vi "KalmanFilter_Predict.vi"(6 "dT_Seconds":dbl=0.02, 10 "U":T2, 11 "in KalmanFilter":T1) -> (0 "Error":bool, 3 "out KalmanFilter":T1)   [LabVIEW 2019, in "Trajectory_Library.lvlib"]
doc: "Creates a new LINEAR SYSTEM data cluster with the specified values. \n\n\nInputs: \n - XXX -- XXX.\n\nOutputs:\n - XXX -- XXX."
uses:
  Trajectory_Library.lvlib
  KALMAN_FILTER.ctl
  <vilib>/Analysis/Matrix/Datatypes/RealMatrix.ctl
  LINEAR_SYSTEM.ctl
  Discretization_DiscretizeAB.vi
  <vilib>/Analysis/baseanly.llb/A x B.vi
  <vilib>/Analysis/baseanly.llb/Real A x B.vi
  <vilib>/Analysis/7linalg.llb/Matrix Exp.vi
  <vilib>/Analysis/7linalg.llb/Real Matrix Exp.vi
  <vilib>/Analysis/Matrix/Numeric/Multiply/Multiply.vi
  <vilib>/Analysis/Matrix/Numeric/Multiply/Multiply - RM,R.vi
  <vilib>/Analysis/Matrix/Numeric/Add/Add.vi
  <vilib>/Analysis/Matrix/Numeric/Add/Add - RM,RM.vi
  <vilib>/Analysis/Matrix/NI_Matrix.lvlib
panel:
  # "<Inputs,1>"
  # "Steady State Gain  \n<States,Outputs>"
  # "State Estimate <Statess,1>"
  # "<States,States>"
  # "<States,Inputs>"
  # "<Outputs,States>"
  # "<Outputs,Inputs>"
  # "Steady State Gain  \n<States,Outputs>"
  # "State Estimate <Statess,1>"
  # "<States,States>"
  # "<States,Inputs>"
  # "<Outputs,States>"
  # "<Outputs,Inputs>"
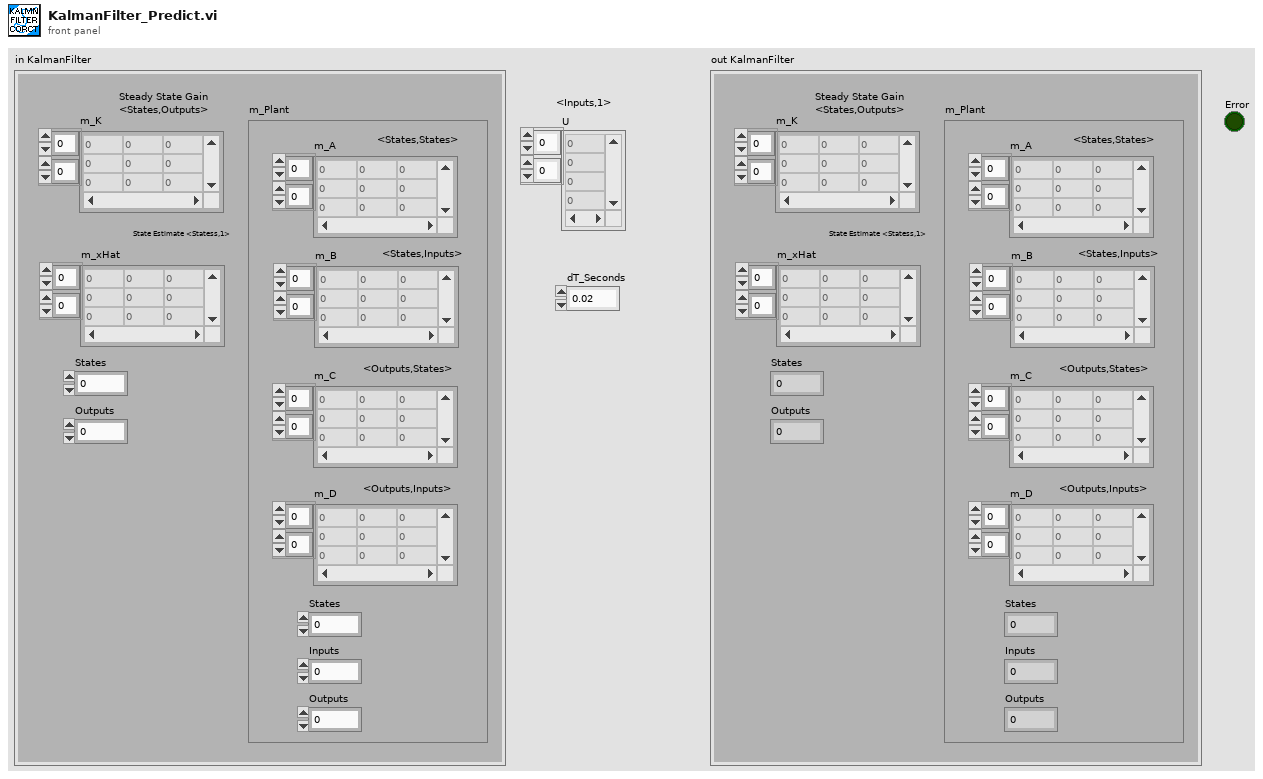
[diagram p1: front panel]
types:
  T1 = typedef "Trajectory_Library.lvlib/KALMAN_FILTER.ctl" = cluster{"m_K":T2, "m_xHat":T2, "States":i32, "Outputs":i32, "m_Plant":T3}
  T2 = typedef "NI_Matrix.lvlib/RealMatrix.ctl" = dbl[][]
  T3 = typedef "Trajectory_Library.lvlib/LINEAR_SYSTEM.ctl" = cluster{"m_A":T2, "m_B":T2, "m_C":T2, "m_D":T2, "States":i32, "Inputs":i32, "Outputs":i32}
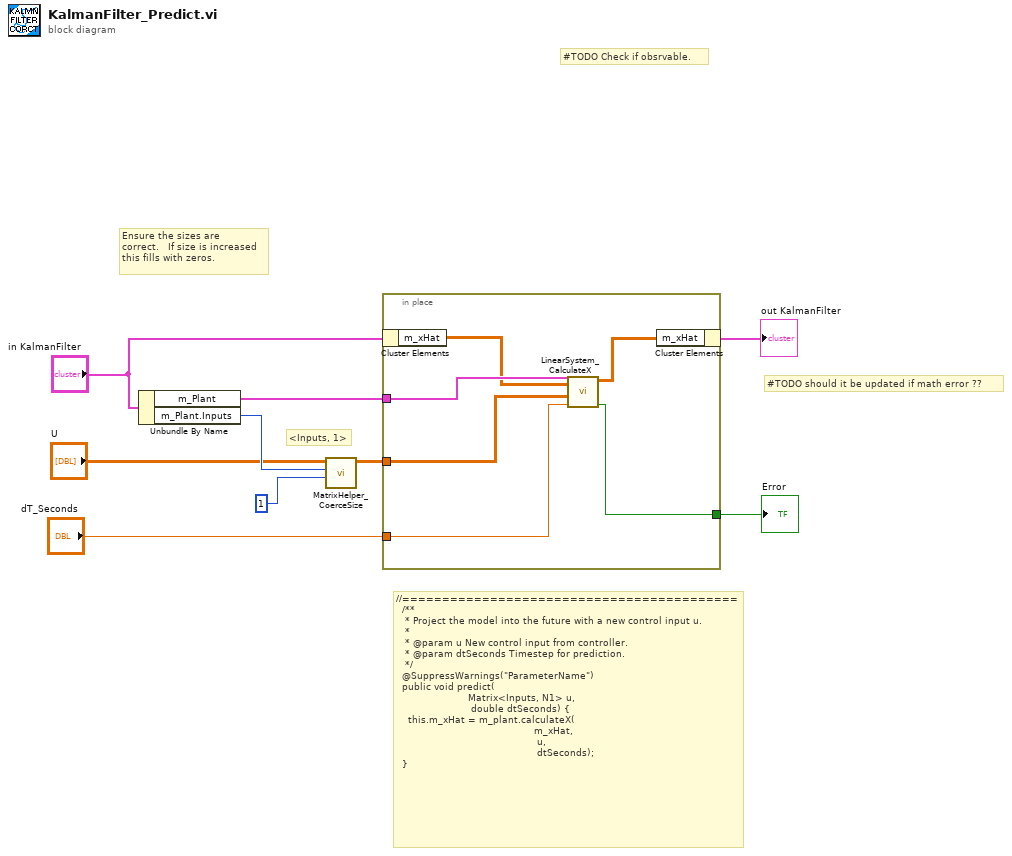
[diagram p0: block diagram]
diagram:
  # "//==========================================\n  /**\n   * Project the model into the future with a new control input u.\n   *\n   * @param u New control input from controller.\n   * @param dtSeconds Timestep for prediction.\n   */\n  @SuppressWarnings(\"ParameterName\")\n  public void predict(\n                        Matrix<Inputs, N1> u, \n                         double dtSeconds) {\n    this.m_xHat = m_plant.calculateX(\n                                              m_xHat, \n                                               u, \n                                               dtSeconds);\n  }"
  # "#TODO should it be updated if math error ??"
  # "<Inputs, 1>"
  # "#TODO Check if obsrvable."
  # "Ensure the sizes are\ncorrect.   If size is increased \nthis fills with zeros."
  n1 = Unbundle By Name("in KalmanFilter") -> ("m_Plant"=w7:T3, "m_Plant.Inputs"=w4:i32)
  n2 = call "MatrixHelper_CoerceSize.vi"("Columns"=1 ("y"), "Rows"=w4, "input matrix"="U") -> ("output matrix"=w1:T2)  [unwired: 8 in]
  n3 = in-place {
    in-place-border: w1 -> [w11]
    in-place-border: w7 -> [w15]
    in-place-border: "dT_Seconds" -> [w14]
    in-place-border: [w10] -> w5
    n4 = in-place-cluster #1("in KalmanFilter") -> ("m_xHat"=w13:T2)
    n5 = call "LinearSystem_CalculateX.vi"("dT_Seconds"=w14, "ClampedU"=w11, "X"=w13, "Linearsystem"=w15) -> ("Error"=w10:bool, "X"=w12:T2)  [unwired: 6 in]
    n6 = in-place-cluster #1("m_xHat"=w12) -> (→"out KalmanFilter":T1)
  }
  "Error" <- w5
